vi "SM传输的序列（激活子载波）.vi"() -> ()   [LabVIEW 2018]
panel:
  in  "SM传输的比特（激活子载波）":i32[](array[numeric])
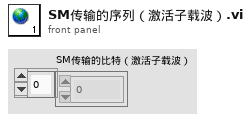
[diagram p1: front panel]
diagram:
